vi "Verileri GUI'ye Gönder.vi"(3 "Uygulanan Değer":dbl, 4 "FD2 C":dbl, 5 "FD2 B":dbl, 6 "FD2 A":dbl, 7 "FD1 C":dbl, 8 "FD1 B":dbl, 9 "FD1 A":dbl, 10 "Limit Deger":dbl, 11 "Ölçüm No":u16) -> ()   [LabVIEW 2014]
uses:
  VeriPaylasim_Globali.vi
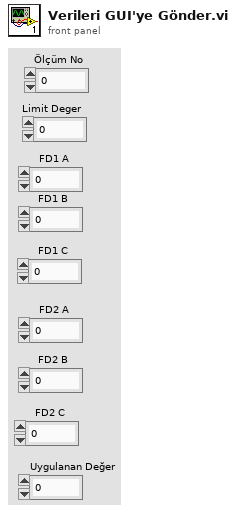
[diagram p1: front panel]
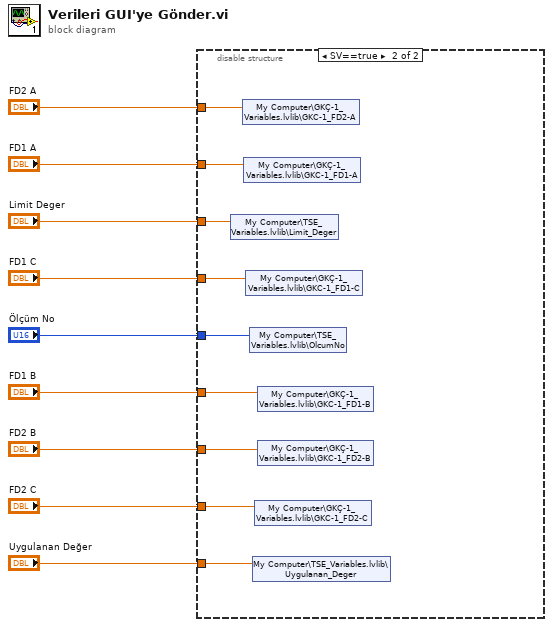
[diagram p0: block diagram]
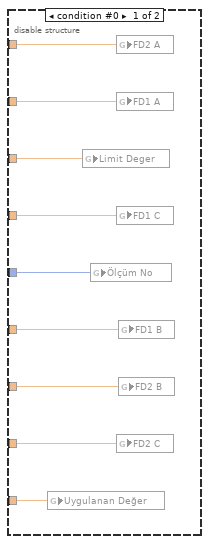
[diagram p2: hidden frame]
diagram:
  n1 = disable-structure shown="SV==true" {
    disable-tunnel: "FD1 C" -> [w18 w25]
    disable-tunnel: "Limit Deger" -> [w17 w20]
    disable-tunnel: "FD2 A" -> [w16 w24]
    disable-tunnel: "FD1 A" -> [w15 w27]
    disable-tunnel: "Ölçüm No" -> [w14 w21]
    disable-tunnel: "FD1 B" -> [w13 w26]
    disable-tunnel: "FD2 B" -> [w12 w23]
    disable-tunnel: "FD2 C" -> [w11 w22]
    disable-tunnel: "Uygulanan Değer" -> [w10 w19]
    frame condition #0 {
      n2 = global write "VeriPaylasim_Globali.vi" "Uygulanan Değer"(w10) -> ()
      n3 = global write "VeriPaylasim_Globali.vi" "Limit Deger"(w17) -> ()
      n4 = global write "VeriPaylasim_Globali.vi" "Ölçüm No"(w14) -> ()
      n5 = global write "VeriPaylasim_Globali.vi" "FD2 A"(w16) -> ()
      n6 = global write "VeriPaylasim_Globali.vi" "FD1 A"(w15) -> ()
      n7 = global write "VeriPaylasim_Globali.vi" "FD1 C"(w18) -> ()
      n8 = global write "VeriPaylasim_Globali.vi" "FD2 C"(w11) -> ()
      n9 = global write "VeriPaylasim_Globali.vi" "FD1 B"(w13) -> ()
      n10 = global write "VeriPaylasim_Globali.vi" "FD2 B"(w12) -> ()
    }
    frame condition #1 (active) {
      n11 = shared-variable "My Computer\\TSE_Variables.lvlib\\Limit_Deger"(w20) -> ()  [unwired: 1 in, 1 out]
      n12 = shared-variable "My Computer\\GKÇ-1_Variables.lvlib\\GKC-1_FD2-A"(w24) -> ()  [unwired: 1 in, 1 out]
      n13 = shared-variable "My Computer\\GKÇ-1_Variables.lvlib\\GKC-1_FD1-A"(w27) -> ()  [unwired: 1 in, 1 out]
      n14 = shared-variable "My Computer\\GKÇ-1_Variables.lvlib\\GKC-1_FD1-C"(w25) -> ()  [unwired: 1 in, 1 out]
      n15 = shared-variable "My Computer\\TSE_Variables.lvlib\\OlcumNo"(w21) -> ()  [unwired: 1 in, 1 out]
      n16 = shared-variable "My Computer\\TSE_Variables.lvlib\\Uygulanan_Deger"(w19) -> ()  [unwired: 1 in, 1 out]
      n17 = shared-variable "My Computer\\GKÇ-1_Variables.lvlib\\GKC-1_FD2-C"(w22) -> ()  [unwired: 1 in, 1 out]
      n18 = shared-variable "My Computer\\GKÇ-1_Variables.lvlib\\GKC-1_FD1-B"(w26) -> ()  [unwired: 1 in, 1 out]
      n19 = shared-variable "My Computer\\GKÇ-1_Variables.lvlib\\GKC-1_FD2-B"(w23) -> ()  [unwired: 1 in, 1 out]
    }
  }
